vi "move.vi"(8 "error in (no error)":errorcluster, 10 "translation vector":refnum<class "SpaceVector.lvclass">, 11 "Box in":refnum<class "Box.lvclass">) -> (0 "error out":errorcluster, 3 "Box out":refnum<class "Box.lvclass">)   [LabVIEW 2010, in "Box.lvclass"]
uses:
  Box.lvclass
  SpaceVector/SpaceVector/SpaceVector.lvclass
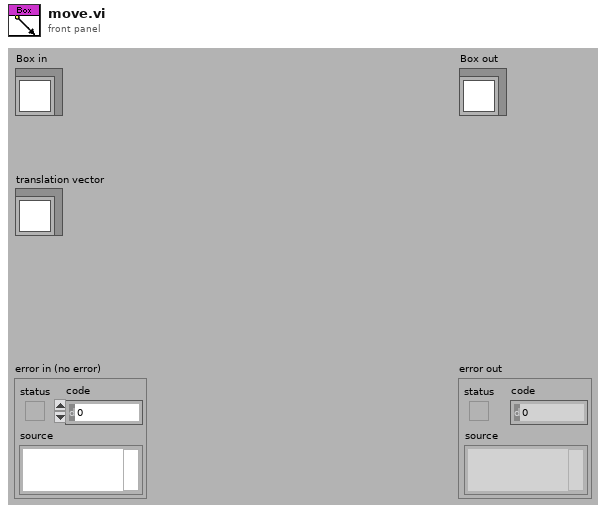
[diagram p1: front panel]
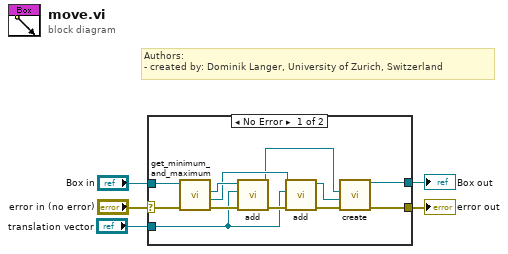
[diagram p0: block diagram]
diagram:
  # "Authors: \n- created by: Dominik Langer, University of Zurich, Switzerland"
  n1 = case shown="No Error" "error in (no error)" {
    selector: "error in (no error)" -> [w16 w19]
    tunnel: [w7 w19] -> w4
    tunnel: [w6 w18] -> w2
    tunnel: "Box in" -> [w17 w18]
    tunnel: "translation vector" -> [w11 _]
    frame No Error {
      n2 = call "get_minimum_and_maximum.vi"("error in (no error)"=w16, "Box in"=w17) -> ("error out"=w14:errorcluster, "maximum"=w13:refnum<class "SpaceVector.lvclass">, "minimum"=w15:refnum<class "SpaceVector.lvclass">)  [unwired: 6 in, 1 out]
      n3 = call "add.vi"("error in (no error)"=w14, "vector to be added"=w11, "SpaceVector in"=w15) -> ("error out"=w12:errorcluster, "SpaceVector out"=w10:refnum<class "SpaceVector.lvclass">)  [unwired: 7 in]
      n4 = call "add.vi"("error in (no error)"=w12, "vector to be added"=w11, "SpaceVector in"=w13) -> ("error out"=w8:errorcluster, "SpaceVector out"=w9:refnum<class "SpaceVector.lvclass">)  [unwired: 7 in]
      n5 = call "create.vi"("error in (no error)"=w8, "maximum"=w9, "minimum"=w10) -> ("error out"=w7:errorcluster, "Box out"=w6:refnum<class "Box.lvclass">)  [unwired: 7 in]
    }
    frame Error {
    }
  }
  "error out" <- w4
  "Box out" <- w2
